vi "WPI_CameraGet Enum Appearance Property.vi"(8 "error in (no error)":errorcluster, 9 "Strings":string[](array[string]), 10 "Property Name":string, 11 "CameraDevRef":T1) -> (0 "error out":errorcluster, 2 "Enum Int Value":i32, 3 "CameraDevRef out":T1)   [LabVIEW 2017]
doc: "This software is licensed. Open the labview\\readme\\WPI Robotics Library Open Source License.txt file for more information."
uses:
  <vilib>/Rock Robotics/WPI/Camera/WPI_CameraDevRef.ctl
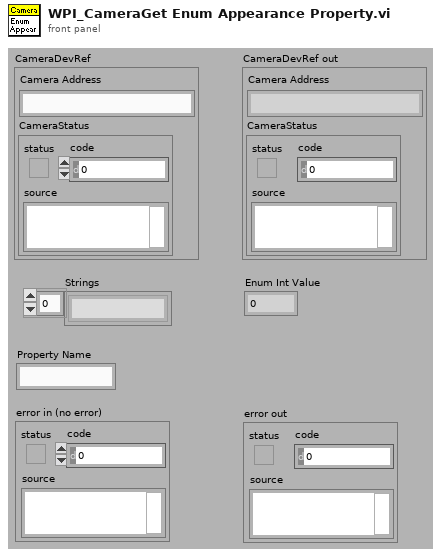
[diagram p1: front panel]
types:
  T1 = typedef "WPI_CameraDevRef.ctl" = cluster{"Camera Address":string, "CameraStatus":errorcluster}
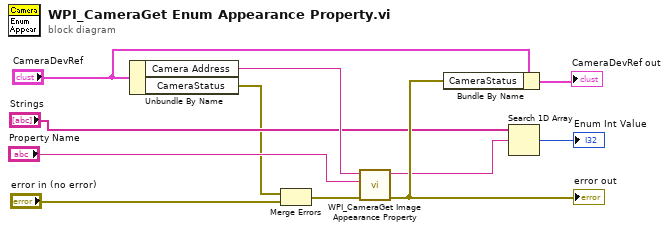
[diagram p0: block diagram]
diagram:
  n1 = Unbundle By Name("CameraDevRef") -> ("Camera Address"=w8:string, "CameraStatus"=w3:errorcluster)
  n2 = Merge Errors(w3, "error in (no error)") -> (w1:errorcluster)
  n3 = call <vilib>:"WPI_CameraGet Image Appearance Property.vi"("error in (no error)"=w1, "Prop String"="Property Name", "address"=w8) -> ("error out"=w10:errorcluster, "Value"=w6:string)  [unwired: 1 in, 6 out]
  "error out" <- w10
  n4 = Bundle By Name(cluster="CameraDevRef", "CameraStatus"=w10) -> (→"CameraDevRef out":T1)
  n5 = Search 1D Array(1D array="Strings", element=w6) -> (index of element=→"Enum Int Value":i32)  [unwired: 1 out]
